vi "Test Bench v12 - TDMS.vi"() -> ()   [LabVIEW 2022 SP3]
uses:
  WhiteNoise.ctl
  <vilib>/Utility/error.llb/DialogType.ctl
  <vilib>/DAQmx/read.llb/DAQmx Read (Analog 1D DBL 1Chan NSamp).vi
  <vilib>/DAQmx/write.llb/DAQmx Write (Analog 2D DBL NChan NSamp).vi
  <vilib>/DAQmx/create/channels.llb/DAQmx Create Channel (AI-Acceleration-Accelerometer).vi
  <vilib>/DAQmx/create/channels.llb/DAQmx Create Channel (AO-Voltage-Basic).vi
  <vilib>/DAQmx/configure/timing.llb/DAQmx Timing (Sample Clock).vi
  <vilib>/DAQmx/miscellaneous.llb/DAQmx Fill In Error Info.vi
  <resource>/objmgr/daqmx.rc
  <vilib>/measure/NI_MABase.lvlib
  <vilib>/DAQmx/configure/task.llb/DAQmx Configure Logging (TDMS).vi
panel:
  in  "Folder to save file to":path=path "C:/Users/LAV-UFSC/OneDrive - UFSC/Documents-LAV-UFSC/LAV-TCC/Dados-Experimentos/Dados-Bancada-LABVIEW"
  out "Waveform Chart 3":dbl[](graph)
  out "Waveform Chart":dynamicdata(graph)
  in  "Log Raw\nData":bool
  in  "Accel. 2":bool
  in  "Start\nReading":bool=TRUE
  out "New file path":path
  in  "Signal Output Control":enum32{"White Noise", "Harmonic"}(tab)
  in  "White Noise\nParameters":T2={"Seed"=0.0, "Standard Deviation"=0.2, "Reset"=FALSE, "Iterator"=1.0, "Seed"=-1, "Stop 4"=FALSE, "Lower Cut-Off"=5.0, "Upper Cut-Off"=350.0} {"Upper Cut-Off" min=5.0 max=350.0 step=10.0; "Lower Cut-Off" min=5.0 max=350.0 step=10.0; "Standard Deviation" min=0.001 max=1.5 step=0.05 format="%0.2p"}
  out "dt White Noise":dbl
  in  "Hamonic\nParameters":T3={"Waveform Type"=0, "Frequency"=10.0, "Amplitude"=0.25, "Stop 4"=FALSE} {"Frequency" min=5.0 max=350.0 step=10.0 format="%0.2p"; "Waveform Type" items=["Sine Wave", "Triangle Wave", "Square Wave", "Sawtooth Wave"]; "Amplitude" min=0.001 max=0.3 step=0.05 format="%0.2p"}
  out "dt Harmonic":dbl
  in  "Start\nOutput":bool=TRUE
  # "Filter"
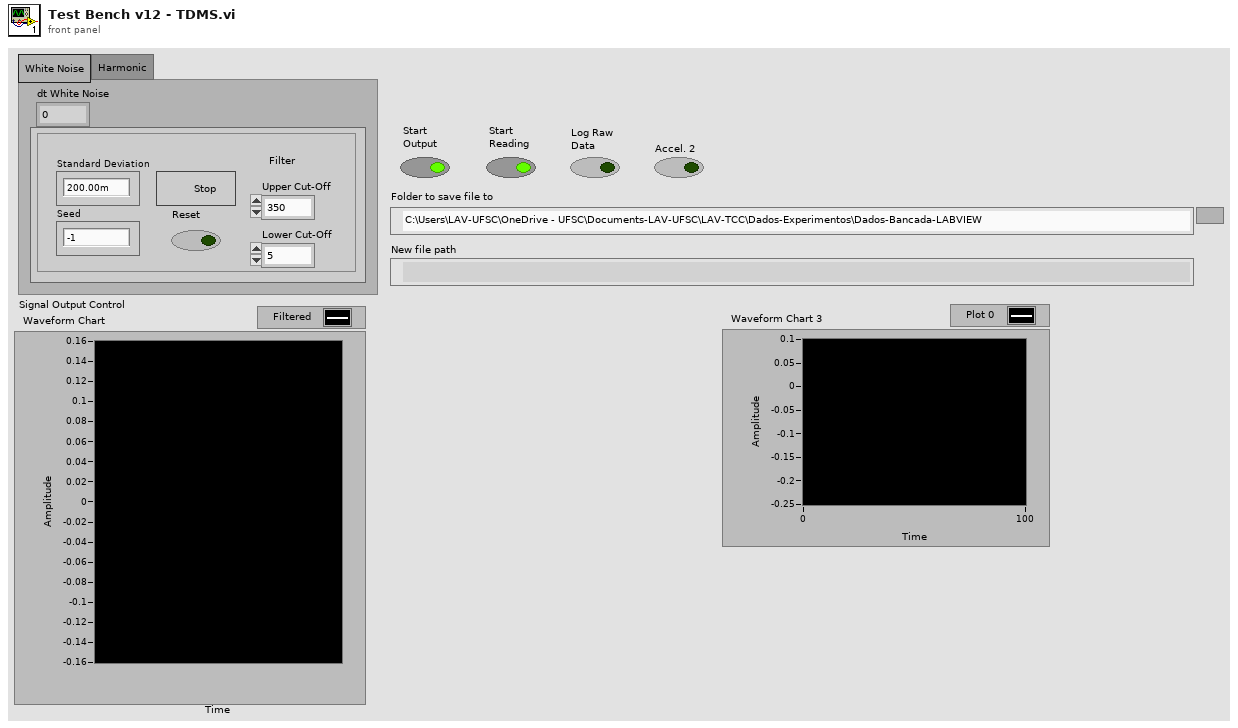
[diagram p1: front panel]
types:
  T1 = typedef "WhiteNoise.ctl" = dbl
  T2 = cluster{"Seed":T1, "Standard Deviation":dbl, "Reset":bool, "Iterator":dbl, "Seed":i8, "Stop 4":bool, "Lower Cut-Off":dbl, "Upper Cut-Off":dbl}
  T3 = cluster{"Waveform Type":u16, "Frequency":dbl, "Amplitude":dbl, "Stop 4":bool}
  T4 = typedef "DialogType.ctl" = u16
  T5 = enum16{"open", "open or create", "create or replace", "create", "open (read-only)"}
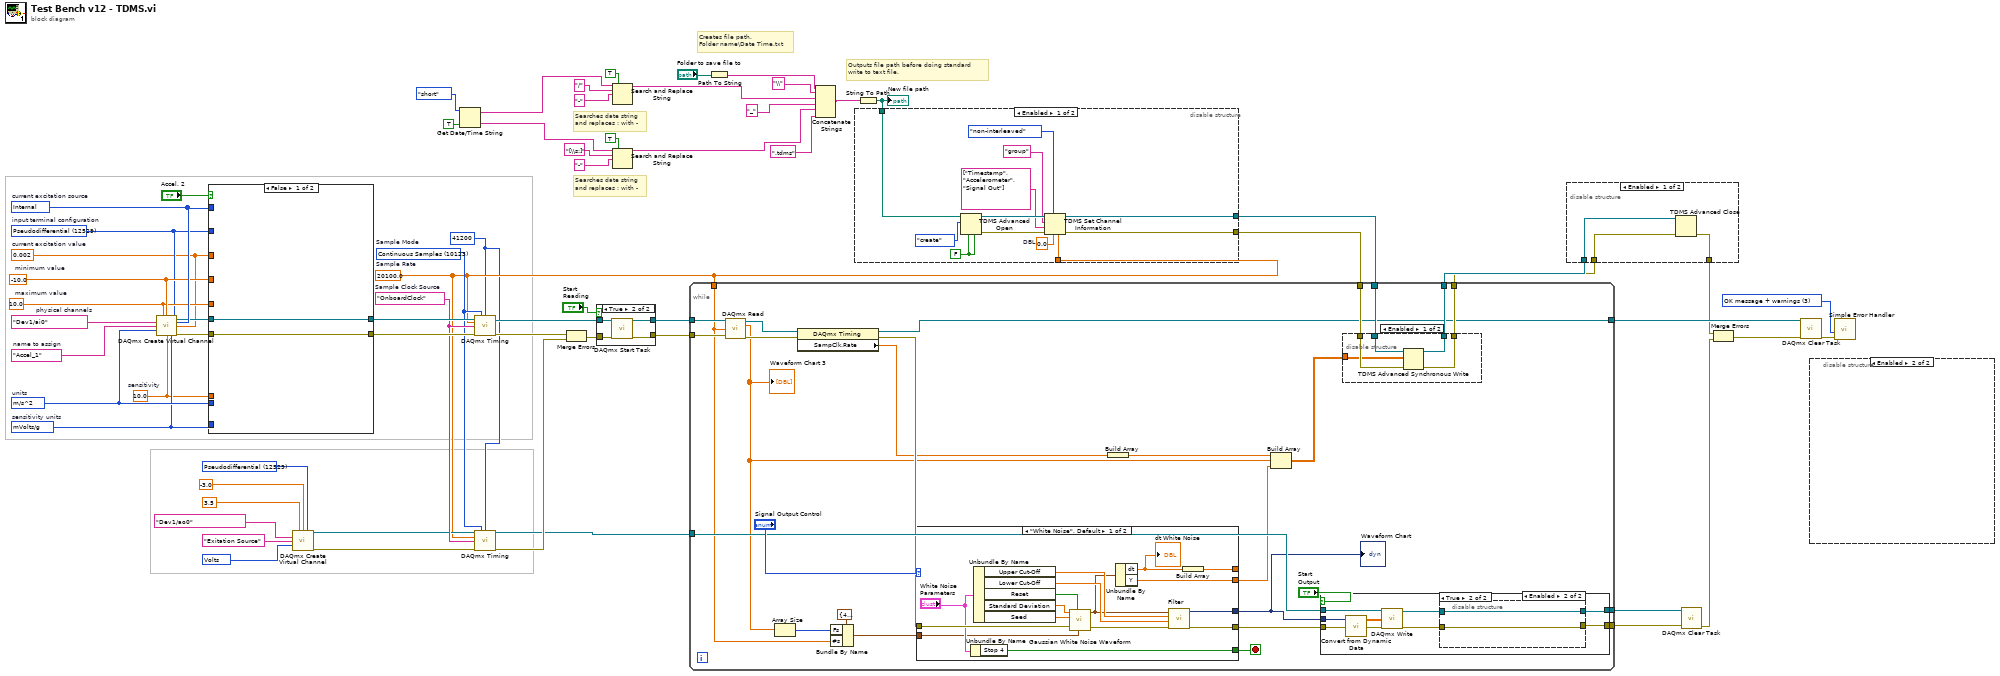
[diagram p0: block diagram]
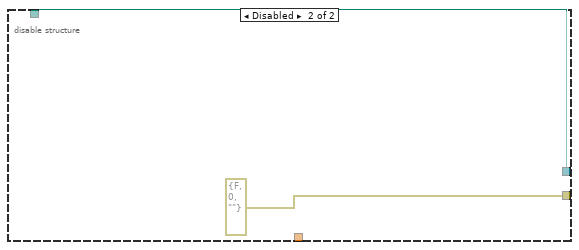
[diagram p2: hidden frame]
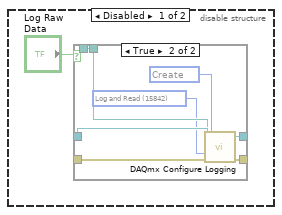
[diagram p4: hidden frame]
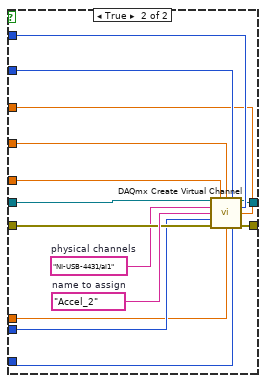
[diagram p6: hidden frame]
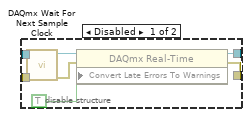
[diagram p10: hidden frame]
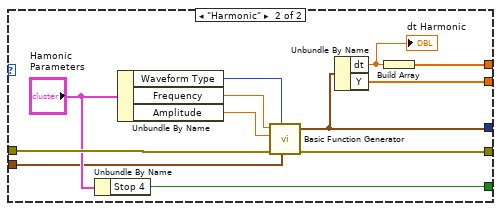
[diagram p11: hidden frame]
diagram:
  w6 = 41200
  w43 = T4 3 items=["no dialog", "OK message", "continue or stop message", "OK message + warnings", "continue/stop + warnings"] ("type of dialog (OK msg:1)")
  w53 = 12529 items=["Default"=-1, "RSE"=10083, "Differential"=10106, "Pseudodifferential"=12529] ("output terminal configuration")
  w51 = 10348 items=["Volts"=10348, "From Custom Scale"=10065] ("units")
  w57 = 12509 items=["mVolts/g"=12509, "Volts/g"=12510]  # sensitivity units
  w47 = 10.0  # sensitivity
  w56 = 0.002  # current excitation value
  w64 = 10200 items=["Internal"=10200, "External"=10167, "None"=10230]  # current excitation source
  w58 = tag "Dev1/ai0"  # physical channels
  w44 = tag "OnboardClock"  # Sample Clock Source
  w7 = 20100.0  # Sample Rate
  w42 = 10123 items=["Finite Samples"=10178, "Continuous Samples"=10123, "Hardware Timed Single Point"=12522]  # Sample Mode
  w60 = 12529 items=["default"=-1, "RSE"=10083, "NRSE"=10078, "Differential"=10106, "Pseudodifferential"=12529]  # input terminal configuration
  w63 = -10.0  # minimum value
  w62 = 10.0  # maximum value
  w66 = "Accel_1"  # name to assign
  w61 = 12470 items=["g"=10186, "m/s^2"=12470, "in/s^2"=12471, "From Custom Scale"=10065]  # units
  # "Searches date string\nand replaces : with -"
  # "Searches date string\nand replaces : with -"
  # "Creates file path.\nFolder name\\Date Time.txt"
  # "Outputs file path before doing standard\nwrite to text file."
  n1 = call-poly <vilib>:"DAQmx Create Virtual Channel.vi"("maximum value"=w62, "minimum value"=w63, "input terminal configuration"=w60, "physical channels"=w58, "current excitation source"=w64, "name to assign"=w66, "current excitation value"=w56, "units"=w61, "sensitivity"=w47, "sensitivity units"=w57) -> ("task out"=w59:refnum<k21>, "error out"=w65:errorcluster)  [unwired: 4 in]
  n2 = case shown="False" "Accel. 2" {
    tunnel: w65 -> [w68 w81]
    tunnel: w64 -> [_ w80]
    tunnel: w63 -> [_ w79]
    tunnel: w62 -> [_ w78]
    tunnel: w61 -> [_ w77]
    tunnel: w60 -> [_ w76]
    tunnel: w59 -> [w67 w75]
    tunnel: w57 -> [_ w73]
    tunnel: w56 -> [_ w72]
    tunnel: w47 -> [_ w71]
    tunnel: [w68 w70] -> w46
    tunnel: [w67 w69] -> w45
    frame False {
    }
    frame True {
      w74 = tag "NI-USB-4431/ai1"  # physical channels
      w82 = "Accel_2"  # name to assign
      n3 = call-poly <vilib>:"DAQmx Create Virtual Channel.vi"("task in"=w75, "maximum value"=w78, "minimum value"=w79, "input terminal configuration"=w76, "physical channels"=w74, "current excitation source"=w80, "name to assign"=w82, "current excitation value"=w72, "units"=w77, "error in"=w81, "sensitivity"=w71, "sensitivity units"=w73) -> ("task out"=w69:refnum<k21>, "error out"=w70:errorcluster)  [unwired: 2 in]
    }
  }
  n4 = call-poly <vilib>:"DAQmx Create Virtual Channel.vi"("maximum value"=3.5, "minimum value"=-3.0, "output terminal configuration"=w53, "physical channels"=tag "Dev1/ao0", "name to assign"="Exitation Source", "units"=w51) -> ("task out"=w40:refnum<k21>, "error out"=w41:errorcluster)  [unwired: 8 in]
  n5 = Get Date/Time String(date format (0)=enum16{"short", "long", "abbreviated"}."short", want seconds? (F)=TRUE) -> (date string=w2:string, time string=w18:string)  [unwired: 1 in]
  n6 = call-poly <vilib>:"DAQmx Timing.vi"("task/channels in"=w45, "sample mode"=w42, "samples per channel"=w6, "rate"=w7, "source"=w44, "error in"=w46) -> ("task out"=w49:refnum<k21>, "error out"=w50:errorcluster)  [unwired: 8 in]
  n7 = call-poly <vilib>:"DAQmx Timing.vi"("task/channels in"=w40, "sample mode"=w42, "samples per channel"=w6, "rate"=w7, "source"=w44, "error in"=w41) -> ("task out"=w38:refnum<k21>, "error out"=w39:errorcluster)  [unwired: 8 in]
  n8 = Merge Errors(w50, w39) -> (w31:errorcluster)
  n9 = case shown="True" "Start\nReading" {
    tunnel: [w83 w85] -> w33
    tunnel: [w84 w86] -> w32
    tunnel: w31 -> [w84 w87]
    tunnel: w49 -> [w83 w88]
    frame False {
    }
    frame True {
      n10 = call <vilib>:"DAQmx Start Task.vi"("task/channels in"=w88, "error in"=w87) -> ("task out"=w85:refnum<k21>, "error out"=w86:errorcluster)  [unwired: 12 in]
    }
  }
  n11 = Search and Replace String(replace all?=TRUE ("replace all? (F)"), input string=w2, search string="/" ("replace string (\"\")"), replace string="-" ("replace string (\"\")")) -> (result string=w1:string)  [unwired: 4 in, 3 out]
  n12 = Search and Replace String(replace all?=TRUE ("replace all? (F)"), input string=w18, search string="[\\s:]" ("replace string (\"\")"), replace string="-" ("replace string (\"\")")) -> (result string=w10:string)  [unwired: 4 in, 3 out]
  n13 = Path To String(path="Folder to save file to") -> (string=w12:string)
  n14 = Concatenate Strings(w12, "\\" ("string"), w1, "_" ("string"), w10, ".tdms" ("string")) -> (w8:string)
  n15 = String To Path(string=w8) -> (path=w28:path)
  "New file path" <- w28
  n16 = disable-structure shown="Enabled" {
    disable-tunnel: w28 -> [w92 w102]
    disable-tunnel: [w91 w102] -> w27
    disable-tunnel: [w90 errorcluster {"status"=FALSE, "code"=0, "source"=""} ("error out")] -> w26
    disable-tunnel: w7 -> [w89 _]
    frame Enabled {
      w93 = 0.0  # DBL
      w95 = FALSE ("enable asynchronous? (T)")
      n17 = TDMS Advanced Open(4:w95, 6:w95, 10:T5."create" ("operation (0:open)"), 11:w92) -> (0:w99:errorcluster, 3:w98:refnum<k34>)  [unwired: 1 in, 1 out]
      n18 = TDMS Set Channel Information(4:w89, 6:w93, 7:enum16{"non-interleaved", "interleaved"}."non-interleaved" ("data layout (0:non-interleaved)"), 8:w99, 9:string[] ["Timestamp", "Accelerometer", "Signal Out"] ("channel name(s)"), 10:"group" ("group name (Untitled)"), 11:w98) -> (0:w90:errorcluster, 3:w91:refnum<k34>)
    }
    frame Disabled {
    }
  }
  n19 = while {
    tunnel: w38 -> [w127]
    tunnel: [w123] -> w37
    tunnel: [w124] -> w36
    tunnel: w33 -> [w126]
    tunnel: w32 -> [w125]
    tunnel: [w115] -> w29
    tunnel: w27 -> [w118]
    tunnel: w26 -> [w121]
    tunnel: [w120] -> w25
    tunnel: [w119] -> w24
    tunnel: w7 -> [w111]
    stop <- w122 stop-if-true
    n20 = call-poly <vilib>:"DAQmx Read.vi"("task/channels in"=w126, "number of samples per channel"=w111, "error in"=w125) -> ("task out"=w116:refnum<k21>, "data"=w105:dbl[], "error out"=w114:errorcluster)  [unwired: 10 in]
    "Waveform Chart 3" <- w105
    n21 = Array Size(array=w105) -> (size(s)=w109:i32)
    n22 = property class="DAQmx Timing"(reference=w116, error in=w114) -> (reference out=w115:refnum<k21>, error out=w113:errorcluster, "SampClk.Rate"=w108:dbl)
    n23 = Bundle By Name(cluster=cluster{"Fs":dbl, "#s":dbl} {"Fs"=41200.0, "#s"=41200.0} ("sampling info"), "Fs"=w109, "#s"=w111) -> (w112:cluster{"Fs":dbl, "#s":dbl})
    n24 = case shown="\"White Noise\", Default" "Signal Output Control" {
      tunnel: w113 -> [w171 w183]
      tunnel: [w168 w182] -> w128
      tunnel: [w170 w180] -> w122
      tunnel: w112 -> [w166 w179]
      tunnel: [w158 w174] -> _
      tunnel: [w157 w173] -> w104
      tunnel: [w156 w172] -> w103
      frame "White Noise", Default {
        n25 = Unbundle By Name("White Noise\nParameters") -> ("Stop 4"=w170:bool)
        n26 = Unbundle By Name("White Noise\nParameters") -> ("Upper Cut-Off"=w162:dbl, "Lower Cut-Off"=w161:dbl, "Reset"=w163:bool, "Standard Deviation"=w164:dbl, "Seed"=w165:T1)
        n27 = call <vilib>:"Gaussian White Noise Waveform.vi"("sampling info"=w166, "reset signal"=w163, "error in (no error)"=w171, "seed"=w165, "standard deviation"=w164) -> ("error out"=w169:errorcluster, "signal out"=w160:waveform(dbl))  [unwired: 5 in]
        n28 = Unbundle By Name(w160) -> ("dt"=w159:dbl, "Y"=w156:dbl[])
        "dt White Noise" <- w159
        n29 = call "Filter"("error in (no error)"=w169, "Lower Cut-Off"=w161, "Upper Cut-Off"=w162, "Signal"=w160) -> ("error out"=w168:errorcluster, "Filtered Signal"=w157:dynamicdata)  [unwired: 6 in]
        n30 = Build Array(w159) -> (w158:dbl[])
      }
      frame "Harmonic" {
        n31 = Unbundle By Name("Hamonic\nParameters") -> ("Stop 4"=w180:bool)
        n32 = Unbundle By Name("Hamonic\nParameters") -> ("Waveform Type"=w178:u16, "Frequency"=w177:dbl, "Amplitude"=w176:dbl)
        n33 = call <vilib>:"Basic Function Generator.vi"("sampling info"=w179, "signal type"=w178, "error in (no error)"=w183, "amplitude"=w176, "frequency"=w177) -> ("error out"=w182:errorcluster, "signal out"=w173:waveform(dbl))  [unwired: 4 in, 1 out]
        n34 = Unbundle By Name(w173) -> ("dt"=w175:dbl, "Y"=w172:dbl[])
        "dt Harmonic" <- w175
        n35 = Build Array(w175) -> (w174:dbl[])
      }
    }
    "Waveform Chart" <- w104
    n36 = Build Array(w108) -> (w106:dbl[])
    n37 = Build Array(w106, w105, w103) -> (w107:dbl[][])
    n38 = case shown="True" "Start\nOutput" {
      tunnel: w128 -> [w137 w146]
      tunnel: w127 -> [w138 w145]
      tunnel: [w137 w141] -> w124
      tunnel: [w138 w142] -> w123
      tunnel: w104 -> [_ w140]
      frame False {
      }
      frame True {
        n39 = call "Convert from Dynamic Data"("Dynamic Data Type"=w140) -> ("Array"=w139:dbl[][])  [unwired: 3 in]
        n40 = call-poly <vilib>:"DAQmx Write.vi"("task/channels in"=w145, "data"=w139, "error in"=w146) -> ("task out"=w144:refnum<k21>, "error out"=w143:errorcluster)  [unwired: 10 in, 1 out]
        n41 = disable-structure shown="Enabled" {
          disable-tunnel: w144 -> [w153 w154]
          disable-tunnel: w143 -> [w152 w155]
          disable-tunnel: [w150 w154] -> w142
          disable-tunnel: [w149 w155] -> w141
          frame Disabled {
            n42 = call <vilib>:"DAQmx Wait For Next Sample Clock.vi"("task/channels in"=w153, "error in"=w152) -> ("task out"=w151:refnum<k21>, "error out"=w148:errorcluster)  [unwired: 11 in, 1 out]
            n43 = property class="DAQmx Real-Time"(reference=w151, error in=w148, "Convert Late Errors To Warnings"=TRUE ("ConvLateErrorsToWarnings")) -> (reference out=w150:refnum<k21>, error out=w149:errorcluster)
          }
          frame Enabled {
          }
        }
      }
    }
    n44 = disable-structure shown="Enabled" {
      disable-tunnel: w121 -> [w134 w136]
      disable-tunnel: [w133 w135] -> w120
      disable-tunnel: [w132 w136] -> w119
      disable-tunnel: w107 -> [w131 _]
      disable-tunnel: w118 -> [w130 w135]
      frame Enabled {
        n45 = TDMS Advanced Synchronous Write(8:w134, 10:w131, 11:w130) -> (0:w132:errorcluster, 3:w133:refnum<k34>)
      }
      frame Disabled {
      }
    }
  }
  n46 = disable-structure shown="Enabled" {
    disable-tunnel: w25 -> [w186 _]
    disable-tunnel: w24 -> [w185 w187]
    disable-tunnel: [w184 w187] -> w21
    frame Enabled {
      n47 = TDMS Advanced Close(8:w185, 11:w186) -> (0:w184:errorcluster)  [unwired: 2 in, 1 out]
    }
    frame Disabled {
    }
  }
  n48 = call <vilib>:"DAQmx Clear Task.vi"("task in"=w37, "error in"=w36) -> ("error out"=w22:errorcluster)  [unwired: 13 in]
  n49 = Merge Errors(w21, w22) -> (w23:errorcluster)
  n50 = call <vilib>:"DAQmx Clear Task.vi"("task in"=w29, "error in"=w23) -> ("error out"=w30:errorcluster)  [unwired: 13 in]
  n51 = disable-structure shown="Enabled" {
    frame Disabled {
      n52 = case shown="True" "Log Raw\nData" {
        tunnel: _ -> [w190 w197]
        tunnel: [w190 w196] -> _
        tunnel: _ -> [_ w194]
        tunnel: [_ w194] -> _
        tunnel: _ -> [w189 w192]
        tunnel: [w189 w193] -> _
        frame False {
        }
        frame True {
          w195 = 15848 items=["Open"=10437, "Open or Create"=15846, "Create or Replace"=15847, "Create"=15848] ("operation")
          w191 = 15842 items=["Off"=10231, "Log"=15844, "Log and Read"=15842] ("logging mode")
          n53 = call-poly <vilib>:"DAQmx Configure Logging.vi"("task/channels in"=w197, "operation"=w195, "file path"=w194, "logging mode"=w191, "error in"=w192) -> ("task out"=w196:refnum<k21>, "error out"=w193:errorcluster)  [unwired: 9 in]
        }
      }
    }
    frame Enabled {
    }
  }
  n54 = call <vilib>:"Simple Error Handler.vi"("type of dialog (OK msg:1)"=w43, "error in (no error)"=w30) -> ()  [unwired: 3 in, 5 out]
